vi "NI VeriStand - Get Channel Data Reference.vi"(8 "error in (no error)":errorcluster, 9 "Access":T3, 10 "Channel Ref in":T1=18446744073709551615 format="%.0x", 11 "Device Ref in":T1=18446744073709551615 format="%.0x") -> (0 "error out":errorcluster, 2 "Channel Data Reference":T2 format="%.0x", 3 "Device Ref out":T1=18446744073709551615 format="%.0x")   [LabVIEW 2020, in "Custom Device API.lvlib"]
doc: "Returns a 32-bit <B>Channel Data Reference</B> to the inline custom device channel specified by <B>Channel Ref in</B>. You can use the reference this VI returns with the Get Channel Value by Data Reference and Set Channel Value by Data Reference VIs."
uses:
  <vilib>/NI VeriStand/Custom Device API/Custom Device API.lvlib
  <vilib>/NI VeriStand/Custom Device API/Custom Device Item Ref.ctl
  <vilib>/NI VeriStand/Custom Device API/Data Access Type.ctl
  <vilib>/NI VeriStand/Custom Device API/Data Reference.ctl
  b85ba52d-5a32-4fc7-a674-bcccb96345a3.vi
  <vilib>/NI VeriStand/Custom Device API/Custom Device Offline Path.vi
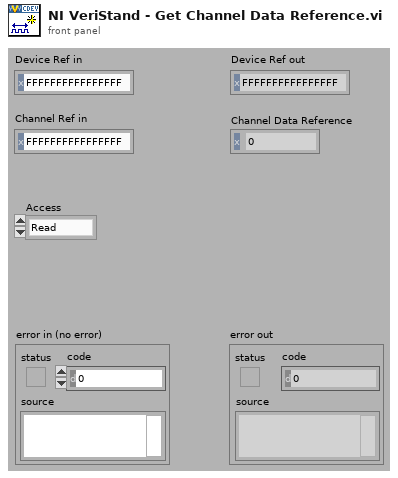
[diagram p1: front panel]
types:
  T1 = typedef "Custom Device API.lvlib/Custom Device Item Ref.ctl" = u64
  T2 = typedef "Custom Device API.lvlib/Data Reference.ctl" = i32
  T3 = typedef "Custom Device API.lvlib/Data Access Type.ctl" = enum16{"Read", "Write"}
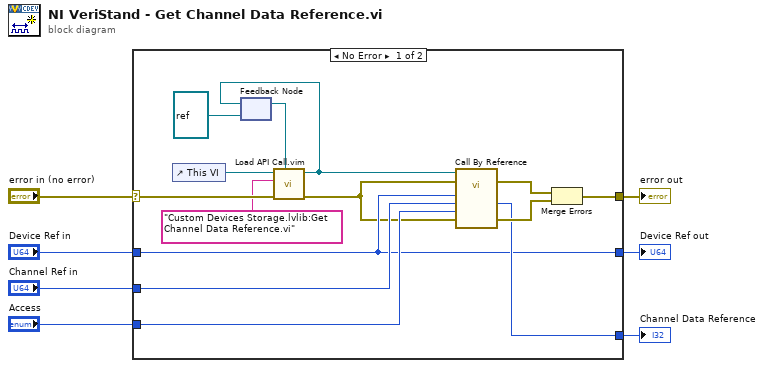
[diagram p0: block diagram]
diagram:
  n1 = case shown="No Error" "error in (no error)" {
    selector: "error in (no error)" -> [w13 w23]
    tunnel: [w20 w23] -> w7
    tunnel: [w16 w22] -> w6
    tunnel: [w19 _] -> w5
    tunnel: "Device Ref in" -> [w16 w22]
    tunnel: "Channel Ref in" -> [w18 _]
    tunnel: "Access" -> [w17 _]
    frame No Error {
      n2 = control-ref of="This VI"() -> (w14:refnum<vi>)
      n3 = feedback #1(refnum<vi> refnum ("type specifier VI Refnum (for type only)")) -> (w15:refnum<vi>)
      n4 = call "Load API Call.vim"("VI reference in"=w15, "error in (no error)"=w13, "VI qualified name"="Custom Devices Storage.lvlib:Get Channel Data Reference.vi", "Caller VI ref"=w14) -> ("error out"=w12:errorcluster, "VI reference"=w11:refnum<vi>)  [unwired: 6 in]
      n5 = feedback-in #1(w11) -> ()
      n6 = call-by-ref "?"(reference=w11, error in=w12, 8:"error in (no error)"=w12, "Access"=w17, "Channel Ref in"=w18, "Device Ref in"=w16) -> (error out=w8:errorcluster, 0:"error out"=w21:errorcluster, "Channel Data Reference"=w19:T2)  [unwired: 5 in, 2 out]
      n7 = Merge Errors(w8, w21) -> (w20:errorcluster)
    }
    frame Error {
    }
  }
  "error out" <- w7
  "Device Ref out" <- w6
  "Channel Data Reference" <- w5
